vi "setConfig.vi"(8 "error in (no error)":errorcluster, 9 "Serial Communication":T1={"Baud Rate"=9600.0, "VISA resource name"="", "Parity"=0, "Data Bits"=8, "Stop Bits"=10, "Flow Control"=0, "termChar"=enum."LF"} {"Flow Control" items=["None", "XON/XOFF", "RTS/CTS", "XON/XOFF & RTS/CTS", "DTR/DSR", "XON/XOFF & DTR/DSR"]; "Stop Bits" items=["1.0"=10, "1.5"=15, "2.0"=20]; "Data Bits" items=["7"=7, "8"=8]; "Parity" items=["None", "Odd", "Even", "Mark", "Space"]}, 10 "Internal Configuration":T3={"IntegrationTime"=0.002, " Input Range "=10.0, "Reading Option (0: Latest)"=0, "Reading Timeout"=600.0, "AVG Filter type"=enum."None", "Filter"=enum."None", "Mode"=enum."Current", "Median Filter"=enum."Active"} {"Input Range" format="%#_10g"}, 11 "Electrometer in":refnum<class "Electrometer.lvclass">) -> (0 "error out":errorcluster, 3 "Electrometer out":refnum<class "Electrometer.lvclass">)   [LabVIEW 2016, in "Electrometer.lvclass"]
uses:
  Electrometer.lvclass
  ElectrometerConfiguration/Controls/internalConfiguration.ctl
  AVG Filter type.ctl
  MED Filter Type.ctl
  Modes.ctl
  ElectrometerConfiguration/Controls/com_conf.ctl
  ts_electrometeruserevents/Typedefs/termChar.ctl
  ElectrometerConfiguration/ElectrometerInternalConfiguration.lvclass
  ElectrometerConfiguration/ElectrometerCOMConfiguration.lvclass
  ts_electrometeruserevents/ConfigurationTC/ConfigurationTypedefs/ConfigurationTypedefs.lvlib
  ts_electrometeruserevents/Typedefs/ElectrometerTypedefs.lvlib
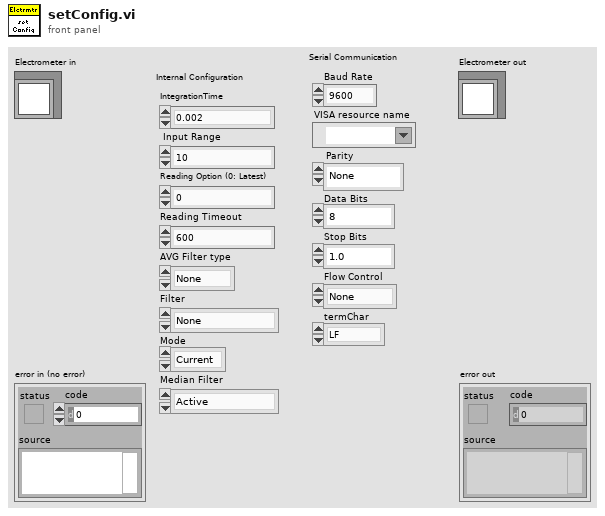
[diagram p1: front panel]
types:
  T1 = typedef "ConfigurationTypedefs.lvlib/com_conf.ctl" = cluster{"Baud Rate":dbl, "VISA resource name":refnum<visa-resource-name>, "Parity":u16, "Data Bits":u16, "Stop Bits":u16, "Flow Control":u16, "termChar":T2}
  T2 = typedef "ElectrometerTypedefs.lvlib/termChar.ctl" = enum16{"CR", "CR+LF", "LF", "LF+CR"}
  T3 = typedef "ConfigurationTypedefs.lvlib/internalConfiguration.ctl" = cluster{"IntegrationTime":dbl, " Input Range ":dbl, "Reading Option (0: Latest)":i32, "Reading Timeout":dbl, "AVG Filter type":T4, "Filter":T5, "Mode":T6, "Median Filter":T5}
  T4 = typedef "Electrometer.lvclass/AVG Filter type.ctl" = enum16{"None", "Scalar", "Advanced"}
  T5 = typedef "Electrometer.lvclass/MED Filter Type.ctl" = enum16{"Active", "None"}
  T6 = typedef "Electrometer.lvclass/Modes.ctl" = enum16{"Current", "Charge"}
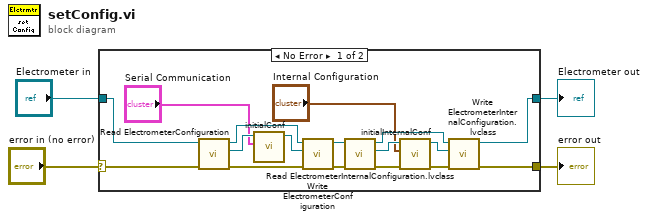
[diagram p0: block diagram]
diagram:
  n1 = case shown="No Error" "error in (no error)" {
    selector: "error in (no error)" -> [w19 w23]
    tunnel: [w5 w23] -> w3
    tunnel: [w6 w22] -> w1
    tunnel: "Electrometer in" -> [w20 w22]
    frame No Error {
      n2 = call "Read ElectrometerConfiguration.vi"("error in (no error)"=w19, "Electrometer in"=w20) -> ("error out"=w16:errorcluster, "ElectrometerConfiguration"=w21:refnum<class "ElectrometerCOMConfiguration.lvclass">, "Electrometer out"=w17:refnum<class "Electrometer.lvclass">)  [unwired: 7 in]
      n3 = call "initialConf.vi"("Serial Communication"="Serial Communication", "ElectrometerConfiguration In"=w21) -> ("ElectrometerConfiguration Out"=w18:refnum<class "ElectrometerCOMConfiguration.lvclass">)  [unwired: 9 in]
      n4 = call-dynamic "Write ElectrometerConfiguration.vi"("error in (no error)"=w16, "ElectrometerConfiguration"=w18, "Electrometer in"=w17) -> ("error out"=w12:errorcluster, "Electrometer out"=w15:refnum<class "Electrometer.lvclass">)  [unwired: 7 in]
      n5 = call-dynamic "Read ElectrometerInternalConfiguration.lvclass.vi"("error in (no error)"=w12, "Electrometer in"=w15) -> ("error out"=w13:errorcluster, "ElectrometerInternalConfiguration.lvclass"=w14:refnum<class "ElectrometerInternalConfiguration.lvclass">, "Electrometer out"=w11:refnum<class "Electrometer.lvclass">)  [unwired: 7 in]
      n6 = call-dynamic "initialInternalConf.vi"("error in (no error)"=w13, "Internal Configuration"="Internal Configuration", "ElectrometerInternalConfiguration in"=w14) -> ("error out"=w9:errorcluster, "ElectrometerInternalConfiguration out"=w10:refnum<class "ElectrometerInternalConfiguration.lvclass">)  [unwired: 7 in]
      n7 = call-dynamic "Write ElectrometerInternalConfiguration.lvclass.vi"("error in (no error)"=w9, "ElectrometerInternalConfiguration.lvclass"=w10, "Electrometer in"=w11) -> ("error out"=w5:errorcluster, "Electrometer out"=w6:refnum<class "Electrometer.lvclass">)  [unwired: 7 in]
    }
    frame Error {
    }
  }
  "error out" <- w3
  "Electrometer out" <- w1
